vi "ArmPathPlannerDemo.vi"() -> ()   [LabVIEW 2018]
uses:
  OperatorControlBox_XControl.xctl
  TypeDefs/GamePiecePosition.ctl
  TypeDefs/ArmPositions.ctl
  TypeDefs/ArmAbsolutePosition.ctl
  TypeDefs/ArmPassThroughParams.ctl
  General/MotionProfiling/TypeDefs/MotionProfileGeneratorParams.ctl
  <vilib>/Rock Robotics/WPI/ThirdParty/Phoenix-LabVIEW/Motor Controller/Controls/CTRE_Phoenix_MotorControl_TrajectoryPointTimeDur.ctl
  TypeDefs/RobotID.ctl
  TypeDefs/ArmTargetPosition.ctl
  TypeDefs/JoystickControls.ctl
  TypeDefs/RobotComponents/RobotMotors.ctl
  <vilib>/Rock Robotics/WPI/MotorControl/WPI_MotorControlDeviceRef.ctl
  <vilib>/Rock Robotics/WPI/MotorControl/WPI_MotorControlType.ctl
  <vilib>/Rock Robotics/SystemInterfaces/DIO/FPGA_DIOPWMChannel.ctl
  <vilib>/Rock Robotics/WPI/PWM/WPI_PWMDeadband.ctl
  <vilib>/Rock Robotics/SystemInterfaces/DIO/FPGA_DIOChannel.ctl
  TypeDefs/ConfigComponents/Config_Robot.ctl
  ArgosLib/Config/ConfigComponents/TypeDefs/Config_Motor.ctl
  <vilib>/Rock Robotics/WPI/ThirdParty/Phoenix-LabVIEW/Motor Controller/Controls/CTRE_Phoenix_MotorControl_NeutralMode.ctl
  <vilib>/Rock Robotics/WPI/ThirdParty/Phoenix-LabVIEW/Motor Controller/Controls/CTRE_Phoenix_MotorControl_LimitSwitchNormal.ctl
  ArgosLib/Config/ConfigComponents/TypeDefs/Config_MotorCtrlType.ctl
  ArgosLib/Config/ConfigComponents/TypeDefs/Config_IMU.ctl
  <vilib>/Rock Robotics/SystemInterfaces/spilib/spi_bus.ctl
  ArgosLib/Config/ConfigComponents/TypeDefs/Config_DigitalIO.ctl
  ArgosLib/Config/ConfigComponents/TypeDefs/Config_PIDParams.ctl
  ArgosLib/Config/ConfigComponents/TypeDefs/Config_SingleSolenoid.ctl
  <vilib>/Rock Robotics/WPI/Solenoid/WPI_SolenoidChannel.ctl
  ArgosLib/Config/ConfigComponents/TypeDefs/Config_MotionMagicParams.ctl
  TypeDefs/ConfigComponents/Config_Dimensions.ctl
  TypeDefs/ArmCoordinate.ctl
  Climber/TypeDefs/ClimberPositionHeights.ctl
  General/MotionProfiling/TypeDefs/TrajectoryPoint.ctl
  ArgosLib/ArgosLib.lvlib
panel:
  in  "OutputTabControl":enum32{"Animation", "Path", "MotionProfiles"}(tab)
  out "Arm Position":cluster{"X":dbl[], "Y":dbl[]}[](graph)=[{"X"=[-15.5, -15.5, -7.0, -7.0, 7.0, 7.0, 15.5, 15.5, 45.5, 45.5, 7.0, 7.0, -7.0, -7.0, -45.5, -45.5, -15.5], "Y"=[0.0, 8.0, 8.0, 21.0, 21.0, 8.0, 8.0, 0.0, 0.0, 90.0, 90.0, 32.0, 32.0, 90.0, 90.0, 0.0, 0.0]}, {"X"=array[361 elements], "Y"=array[361 elements]}, {"X"=array[361 elements], "Y"=array[361 elements]}, {"X"=[0.0, 0.0], "Y"=[44.25, 26.0]}, {"X"=[0.0, 0.0], "Y"=[26.0, 20.0]}, {"X"=[0.0, -11.999996195182016, -11.999996195182016, 0.0], "Y"=[24.5, 24.4904440794712, 27.4904440794712, 27.5]}]
  out "Path":cluster{dbl[], dbl[]}[](graph)=[{array[361 elements], array[361 elements]}, {array[361 elements], array[361 elements]}, {[-15.5, -15.5, -7.0, -7.0, 7.0, 7.0, 15.5, 15.5, 45.5, 45.5, 7.0, 7.0, -7.0, -7.0, -45.5, -45.5, -15.5], [0.0, 8.0, 8.0, 21.0, 21.0, 8.0, 8.0, 0.0, 0.0, 90.0, 90.0, 32.0, 32.0, 90.0, 90.0, 0.0, 0.0]}, {[-12.5, -12.478433704418581, -12.402951669883615, -12.251987600813688, -12.003975201627373, -11.637348176743261, -11.141323378370641, -10.51590080650951, -9.761080461159862, -8.876862342321713, -7.863246449995051, -6.669969590682957, -5.189969590682963, -3.643302924016296, -2.05663625734963, -0.4566362573496323, 1.143363742650368, 2.7433637426503723, 4.343363742650376, 5.943363742650379, 7.542132189579336, 9.138056426829323, 10.733980664079322, 12.329904901329314, 13.925829138579315, 15.52175337582931, 17.117677613079312, 18.7136018503293, 20.309526087579293, 21.000000000000004, 20.999999999999996, 20.999999999999996, 20.999999999999993, 20.999999999999996, 21.000000000000004, 21.000000000000004, 21.000000000000004, 21.000000000000004, 21.000000000000004, 21.000000000000004, 21.000000000000004, 21.000000000000004, 21.000000000000004, 21.000000000000004], [17.0, 17.01568457860467, 17.07058060372101, 17.180372653953686, 17.36074530790737, 17.62738314418672, 17.988128452094085, 18.44298123162945, 18.99194148279283, 19.635009205584208, 20.372184400003597, 20.999999999999996, 21.0, 21.0, 21.0, 21.0, 21.0, 21.000000000000004, 20.999999999999996, 20.999999999999996, 21.038769982935307, 21.152900736713708, 21.267031490492112, 21.381162244270516, 21.49529299804892, 21.60942375182732, 21.72355450560572, 21.837685259384124, 21.951816013162524, 21.120098440989317, 19.613431774322653, 18.200098440989308, 16.90676510765598, 15.760098440989307, 15.0, 15.0, 15.0, 15.0, 15.0, 15.0, 15.0, 15.0, 15.0, 15.0]}]
  out "Overall Motion":T1(graph)={0.0, "Trajectory Point Interval (ms)"=40, [[0.0, 0.026666666666668868, 0.120000000000007, 0.30666666666667036, 0.6133333333333397, 1.0666666666666762, 1.6800000000000117, 2.4533333333333425, 3.386666666666679, 4.4800000000000075, 5.733333333333341, 7.081688661341715, 8.561688661341712, 10.108355328008379, 11.695021994675045, 13.295021994675043, 14.895021994675043, 16.495021994675046, 18.095021994675047, 19.695021994675052, 21.29426045671642, 22.894260456716413, 24.494260456716418, 26.094260456716416, 27.694260456716425, 29.294260456716426, 30.894260456716435, 32.49426045671643, 34.09426045671643, 35.1752361010282, 36.68190276769486, 38.095236101028206, 39.38856943436153, 40.535236101028204, 41.295334542017514, 41.295334542017514, 41.295334542017514, 41.295334542017514, 41.295334542017514, 41.295334542017514, 41.295334542017514, 41.295334542017514, 41.295334542017514, 41.295334542017514], [0.0, 0.6666666666667217, 2.3333333333334534, 4.666666666666584, 7.666666666666734, 11.333333333333412, 15.333333333333387, 19.333333333333268, 23.333333333333417, 27.333333333333208, 31.333333333333346, 33.70888320020935, 36.99999999999992, 38.66666666666667, 39.66666666666665, 39.99999999999994, 39.99999999999999, 40.00000000000008, 40.000000000000036, 40.00000000000012, 39.98096155103416, 39.99999999999986, 40.00000000000012, 39.99999999999994, 40.00000000000021, 40.000000000000036, 40.00000000000021, 39.99999999999994, 39.99999999999986, 27.024391107794266, 37.666666666666515, 35.333333333333705, 32.33333333333306, 28.666666666666885, 19.002461024732753, 0.0, 0.0, 0.0, 0.0, 0.0, 0.0, 0.0, 0.0, 0.0], [0.0, 16.666666666668043, 41.66666666666829, 58.33333333332828, 75.00000000000372, 91.66666666666696, 99.99999999999937, 99.99999999999702, 100.00000000000372, 99.99999999999476, 100.00000000000347, 59.38874667190008, 82.2779199947643, 41.66666666666874, 24.999999999999467, 8.333333333332327, 1.2434497875801753e-12, 2.1316282072803006e-12, -1.0658141036401503e-12, 2.1316282072803006e-12, -0.47596122414894637, 0.47596122414237385, 6.572520305780927e-12, -4.440892098500626e-12, 6.750155989720952e-12, -4.440892098500626e-12, 4.440892098500626e-12, -6.750155989720952e-12, -2.1316282072803006e-12, -324.3902223051398, 266.05688897180625, -58.33333333332025, -75.00000000001616, -91.66666666665435, -241.6051410483533, -475.0615256183188, 0.0, 0.0, 0.0, 0.0, 0.0, 0.0, 0.0, 0.0]]}
  out "Arm Shoulder":T1(graph)={0.0, "Trajectory Point Interval (ms)"=40, [[-0.43007813505586256, -0.4296420839132172, -0.42811056304482153, -0.4250223924235489, -0.4198751086410621, -0.41209365055679453, -0.40122632478789805, -0.3869398624770717, -0.36877462030765956, -0.34611168583234253, -0.3181268189017525, -0.2793774438131257, -0.219623853265813, -0.15543715949608483, -0.0882278321456805, -0.019637744370704407, 0.04913734990050419, 0.11745107310899316, 0.18468259919421834, 0.2502690642942215, 0.3141727633602416, 0.37673912272857585, 0.4369342229172807, 0.49448072535404136, 0.5491946894538539, 0.6009772159768075, 0.6498023221382211, 0.6957031748966047, 0.7387583479955007, 0.7371712252132288, 0.7058807841602786, 0.6784767269576032, 0.6549310323374246, 0.6351959881097435, 0.6226707887570674, 0.6226707887570674, 0.6226707887570674, 0.6226707887570674, 0.6226707887570674, 0.6226707887570674, 0.6226707887570674, 0.6226707887570674, 0.6226707887570674, 0.6226707887570674], [0.0, 0.010901278566134709, 0.03828802170989104, 0.07720426553181614, 0.12868209456217, 0.1945364521066889, 0.27168314422241213, 0.3571615577706591, 0.45413105423530303, 0.5665733618829257, 0.6996216732647511, 0.96873437721567, 1.4938397636828171, 1.604667344243204, 1.680233183760108, 1.7147521943744022, 1.7193773567802149, 1.7078430802122242, 1.6807881521306294, 1.6396616275000795, 1.5975924766505014, 1.5641589842083568, 1.5048775047176208, 1.4386625609190171, 1.3678491024953123, 1.294563163073842, 1.220627654035339, 1.1475213189595905, 1.0763793274723987, -0.03967806955679776, -0.782261026323755, -0.685101430066884, -0.5886423655044659, -0.4933761056920255, -0.3131299838169038, 0.0, 0.0, 0.0, 0.0, 0.0, 0.0, 0.0, 0.0, 0.0], [0.0, 0.2725319641533677, 0.6846685785939083, 0.9729060955481275, 1.2869457257588466, 1.6463589386129727, 1.9286673028930805, 2.1369603387061744, 2.424237411616098, 2.8110576911905674, 3.3262077845456344, 6.7278175987729725, 13.127634661678677, 2.770689514009672, 1.8891459879226025, 0.8629752653573519, 0.11562906014531693, -0.2883569141997666, -0.6763732020398705, -1.0281631157637472, -1.0517287712394519, -0.8358373110536166, -1.482036987268398, -1.6553735949650927, -1.7703364605926197, -1.832148485536761, -1.8483877259625747, -1.8276583768937094, -1.778549787179795, -27.901434925729912, -18.56457391917393, 2.4289899064217773, 2.411476614060451, 2.3816564953110104, 4.506153046878042, 7.828249595422595, 0.0, 0.0, 0.0, 0.0, 0.0, 0.0, 0.0, 0.0]]}
  out "Arm Extension":T1(graph)={0.0, "Trajectory Point Interval (ms)"=40, [[29.980201800521623, 29.956956524113412, 29.875643069970817, 29.713228111807556, 29.44702766897723, 29.05497549195633, 28.527442644235364, 27.86729960874173, 27.078556309890278, 26.16670512031852, 25.139226769349754, 24.187827400174566, 23.822222489772315, 23.533723806404836, 23.34078517734665, 23.25448379714171, 23.27809658558894, 23.411290964500196, 23.652215722865584, 23.997626394655185, 24.405838581580717, 24.839083510428015, 25.366024174195292, 25.980960243487978, 26.67780740506135, 27.450328244110118, 28.292324638976435, 29.19778666688754, 30.160998972396772, 31.24087620617458, 32.37221793356851, 33.460385102896645, 34.47683997088334, 35.393141861695746, 36.007811652473414, 36.007811652473414, 36.007811652473414, 36.007811652473414, 36.007811652473414, 36.007811652473414, 36.007811652473414, 36.007811652473414, 36.007811652473414, 36.007811652473414], [0.0, -0.5811319102052792, -2.032836353564882, -4.06037395408152, -6.655011070758121, -9.801304425522517, -13.188321193024155, -16.503575887340816, -19.71858247128635, -22.7962797392939, -25.686958774219182, -23.784984229379713, -9.140122760056268, -7.212467084186969, -4.823465726454668, -2.157534505123504, 0.5903197111807756, 3.3298594727813935, 6.023118959134699, 8.635266794740026, 10.205304673138293, 10.831123221182448, 13.173516594181933, 15.373401732317138, 17.421179039334334, 19.313020976219164, 21.049909871657935, 22.636550697777658, 24.08030763773077, 26.99693084444519, 28.28354318484818, 27.20417923320344, 25.411371699667384, 22.907547270310147, 15.36674476944171, 0.0, 0.0, 0.0, 0.0, 0.0, 0.0, 0.0, 0.0, 0.0], [0.0, -14.52829775513198, -36.29261108399007, -50.68844001291595, -64.86592791691503, -78.65733386910989, -84.67541918754095, -82.88136735791652, -80.37516459863836, -76.94243170018878, -72.26697587313203, 47.54936362098672, 366.1215367330861, 48.19139189673249, 59.72503394330752, 66.64828053327909, 68.69635540760699, 68.48849404001544, 67.33148715883263, 65.30369589013318, 39.25094695995668, 15.645463701103868, 58.55983432498712, 54.997128453380114, 51.19443267542989, 47.29604842212076, 43.42222238596926, 39.66602065299307, 36.093923498827785, 72.91558016786048, 32.165308510074816, -26.984098791118516, -44.8201883384014, -62.59561073393094, -188.52006252171094, -384.16861923604273, 0.0, 0.0, 0.0, 0.0, 0.0, 0.0, 0.0, 0.0]]}
  out "Arm Wrist":T1(graph)={0.0, "Trajectory Point Interval (ms)"=40, [[-1.1399218649441374, -1.1401271167743305, -1.140850840049144, -1.14132230153005, -1.1365047811265363, -1.1178912992924164, -1.0702017132109638, -0.9734500998505116, -0.801776128514992, -0.5257829978420447, -0.10845271313207694, 0.27973404246175215, 0.22672620863261558, 0.178875608022439, 0.1383139859985968, 0.1067322525928331, 0.0851051506059308, 0.07415682103779947, 0.07441631260600232, 0.08653187322417216, 0.1104806304708435, 0.1459394874228916, 0.19394990462002182, 0.2547512366794354, 0.3285998292366029, 0.4155054833836992, 0.5155822451523272, 0.6287266123351376, 0.7548959253420735, 0.8328287747867713, 0.8641192158397215, 0.8915232730423969, 0.9150689676625755, 0.9348040118902565, 0.9473292112429327, 0.9473292112429327, 0.9473292112429327, 0.9473292112429327, 0.9473292112429327, 0.9473292112429327, 0.9473292112429327, 0.9473292112429327, 0.9473292112429327, 0.9473292112429327], [0.0, -0.005131295754828846, -0.018093081870335093, -0.011786537022651089, 0.12043801008784216, 0.4653370458529982, 1.1922396520363143, 2.4187903340113057, 4.291849283387989, 6.899828266823682, 10.433257117749195, 9.704668889845728, -1.3251958457284143, -1.196265015254415, -1.014040550596055, -0.7895433351440921, -0.5406775496725577, -0.27370823920328313, 0.006487289205071162, 0.3028890154542461, 0.5987189311667834, 0.8864714238012023, 1.2002604299282558, 1.5200333014853393, 1.846214813929188, 2.172641353677407, 2.5019190442157, 2.82860917957026, 3.1542328251733975, 1.9483212361174451, 0.782261026323755, 0.685101430066884, 0.5886423655044659, 0.4933761056920255, 0.3131299838169038, 0.0, 0.0, 0.0, 0.0, 0.0, 0.0, 0.0, 0.0, 0.0], [0.0, -0.12828239387072116, -0.32404465288765616, 0.1576636211921001, 3.3056136777623313, 8.6224758941289, 18.1725651545829, 30.663767049374783, 46.82647373441707, 65.19947458589232, 88.33572127313782, -18.214705697586673, -275.74661838935356, 3.2232707618499834, 4.555611616458998, 5.612430386299072, 6.221644636788362, 6.674232761731863, 7.004888210208857, 7.410043156229373, 7.395747892813432, 7.1938123158604705, 7.844725153176338, 7.994321788927089, 8.154537811096219, 8.160663493705473, 8.231942263457325, 8.167253383864004, 8.140591140078435, -30.14778972639881, -29.15150524484225, -2.4289899064217773, -2.411476614060451, -2.3816564953110104, -4.506153046878042, -7.828249595422595, 0.0, 0.0, 0.0, 0.0, 0.0, 0.0, 0.0, 0.0]]}
  in  "InputTabControl":T2(tab)
  in  "stop":bool
  in  "OperatorControlBox":cluster{"OperatorControlBox Buttons":T3}(xcontrol)={"OperatorControlBox Buttons"={"Position_FeederStation"=FALSE, "Position_Depot"=FALSE, "Position_NearRocket_Low"=FALSE, "Position_NearRocket_Mid"=FALSE, "Position_NearRocket_High"=FALSE, " Position_FarRocket_Low"=FALSE, "Position_FarRocket_Mid"=FALSE, "Position_FarRocket_High"=FALSE, "Mode_Hatch"=FALSE, "Mode_Cargo"=TRUE, "Side_Left"=TRUE, "Side_Right"=FALSE, "Climb"=FALSE, "Switch1_Left"=TRUE, "Switch1_Right"=FALSE, "Switch2_Left"=TRUE, "Switch2_Right"=FALSE, "Button1"=FALSE, "Button2"=FALSE, "Button3"=FALSE, "Button4"=FALSE, "Position_CargoShip"=FALSE}}
  in  "Game Piece Position":T4={"Hatch Forward"={"FeederStation"={"X (in)"=13.0, "Y (in)"=18.0, "Wrist (rad)"=1.8}, "Low"={"X (in)"=14.0, "Y (in)"=19.0, "Wrist (rad)"=1.7}, "Mid"={"X (in)"=16.0, "Y (in)"=52.0, "Wrist (rad)"=1.57}, "High"={"X (in)"=11.0, "Y (in)"=75.0, "Wrist (rad)"=1.57}, "FloorIntake"={"X (in)"=-12.5, "Y (in)"=17.0, "Wrist (rad)"=-1.57}, "CargoShip"={"X (in)"=9.0, "Y (in)"=19.0, "Wrist (rad)"=1.8}}, "Hatch Reverse"={"FeederStation"={"X (in)"=-16.0, "Y (in)"=24.0, "Wrist (rad)"=-1.57}, "Low"={"X (in)"=-15.0, "Y (in)"=23.0, "Wrist (rad)"=-1.75}, "Mid"={"X (in)"=-16.0, "Y (in)"=52.0, "Wrist (rad)"=-1.57}, "High"={"X (in)"=-9.0, "Y (in)"=79.0, "Wrist (rad)"=-1.7}, "FloorIntake"={"X (in)"=-12.5, "Y (in)"=17.0, "Wrist (rad)"=-1.57}, "CargoShip"={"X (in)"=-11.0, "Y (in)"=24.0, "Wrist (rad)"=-1.57}}, "Cargo Forward"={"FeederStation"={"X (in)"=-12.5, "Y (in)"=17.0, "Wrist (rad)"=-1.57}, "Low"={"X (in)"=13.0, "Y (in)"=32.0, "Wrist (rad)"=2.2}, "Mid"={"X (in)"=9.0, "Y (in)"=60.0, "Wrist (rad)"=2.2}, "High"={"X (in)"=12.0, "Y (in)"=70.0, "Wrist (rad)"=1.57}, "FloorIntake"={"X (in)"=21.0, "Y (in)"=15.0, "Wrist (rad)"=1.57}, "CargoShip"={"X (in)"=16.0, "Y (in)"=52.0, "Wrist (rad)"=1.57}}, "Cargo Reverse"={"FeederStation"={"X (in)"=-16.0, "Y (in)"=25.5, "Wrist (rad)"=-1.57}, "Low"={"X (in)"=-16.0, "Y (in)"=25.5, "Wrist (rad)"=-1.2}, "Mid"={"X (in)"=-16.0, "Y (in)"=52.0, "Wrist (rad)"=-1.2}, "High"={"X (in)"=-9.0, "Y (in)"=78.0, "Wrist (rad)"=-1.4}, "FloorIntake"={"X (in)"=-18.0, "Y (in)"=15.0, "Wrist (rad)"=0.0}, "CargoShip"={"X (in)"=-18.0, "Y (in)"=50.0, "Wrist (rad)"=-1.0}}, "Hold"={"X (in)"=0.0, "Y (in)"=26.0, "Wrist (rad)"=0.0}}
  in  "Arm MotionProfileParams":T7={"Trajectory Point Interval (ms)"=40, "Maximum Travel Speed (units/s)"=40.0, "Velocity Ramp Time (ms)"=400.0, "Acceleration Ramp Time (ms)"=200.0} {"Acceleration Ramp Time (ms)" min=1.0; "Velocity Ramp Time (ms)" min=1.0; "Maximum Travel Speed (units/s)" min=0.0; "Trajectory Point Interval (ms)" items=["TrajectoryDuration_0ms"=0, "TrajectoryDuration_5ms"=5, "TrajectoryDuration_10ms"=10, "TrajectoryDuration_20ms"=20, "TrajectoryDuration_30ms"=30, "TrajectoryDuration_40ms"=40, "TrajectoryDuration_50ms"=50, "TrajectoryDuration_100ms"=100]}
  in  "Arm Pass Through Params":T9={"Pass Through Length (in)"=14.0, "Pass Through Min Height (in)"=21.0, "Pass Through Max Height (in)"=32.0, "Pass Through Wrist Angle (rad)"=0.0}
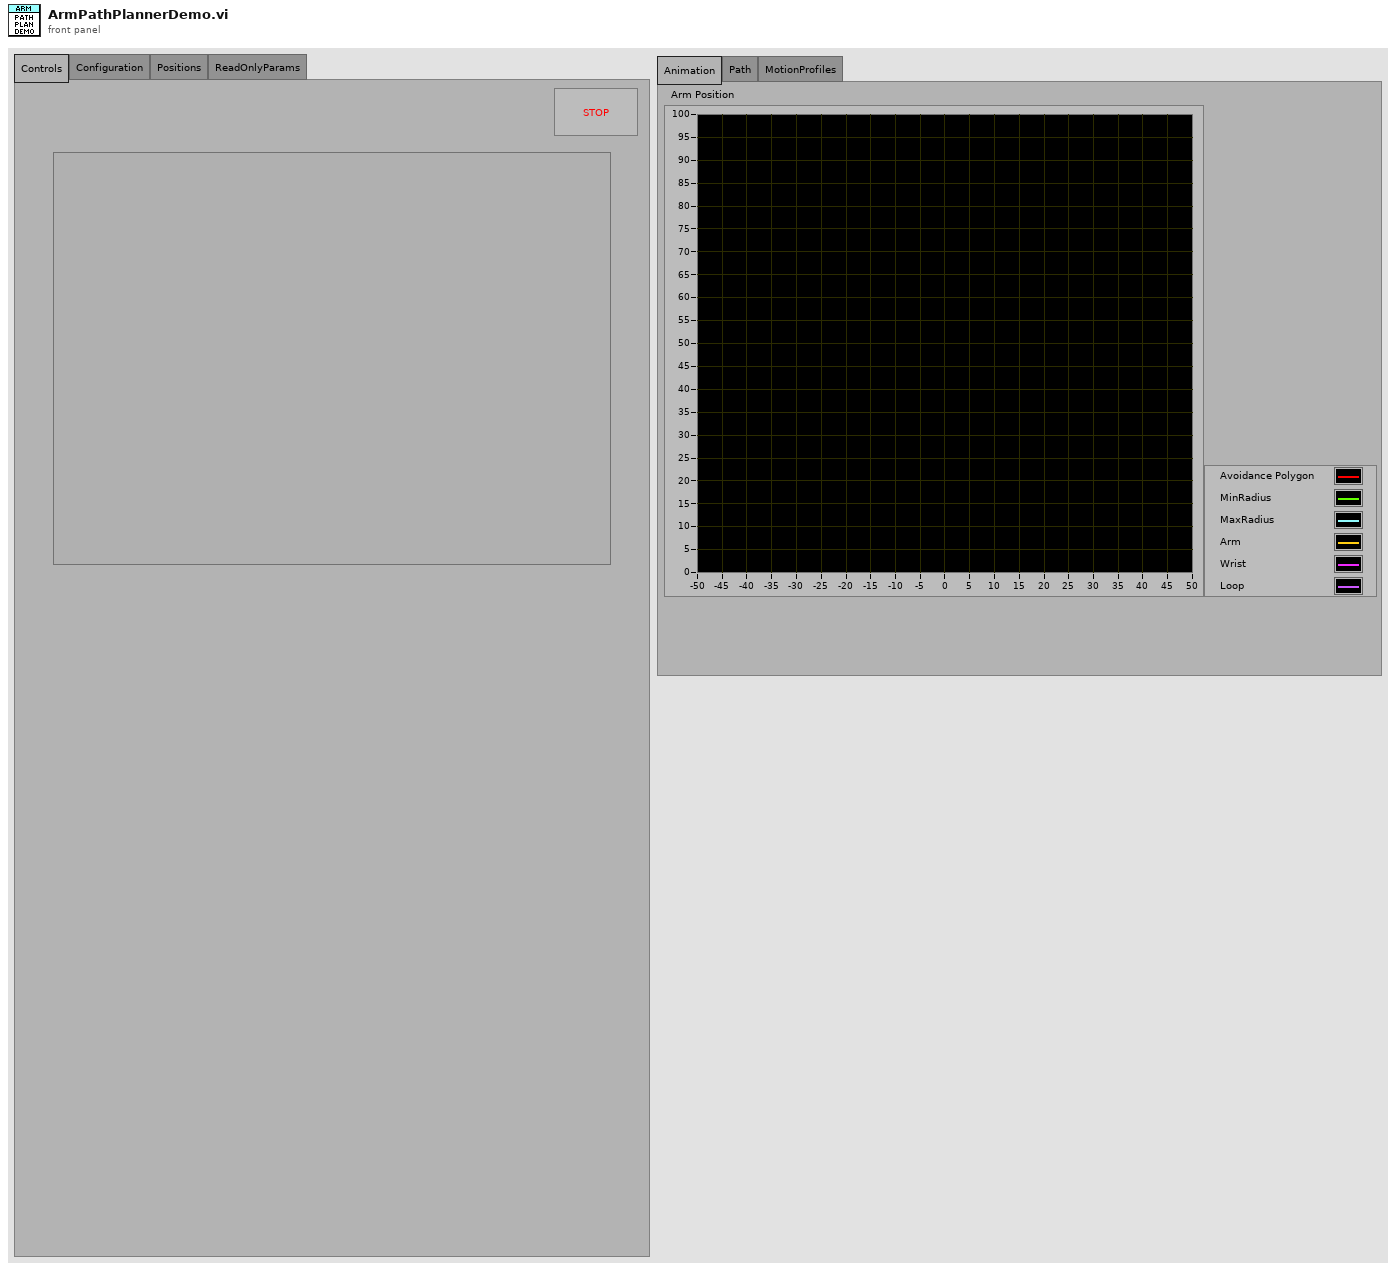
[diagram p1: front panel]
types:
  T1 = cluster{dbl, "Trajectory Point Interval (ms)":i32, dbl[][]}
  T2 = enum32{"Controls", "Configuration", "Positions", "ReadOnlyParams"}
  T3 = typedef "OperatorControlBoxButtons_Type.ctl" = cluster{"Position_FeederStation":bool, "Position_Depot":bool, "Position_NearRocket_Low":bool, "Position_NearRocket_Mid":bool, "Position_NearRocket_High":bool, " Position_FarRocket_Low":bool, "Position_FarRocket_Mid":bool, "Position_FarRocket_High":bool, "Mode_Hatch":bool, "Mode_Cargo":bool, "Side_Left":bool, "Side_Right":bool, "Climb":bool, "Switch1_Left":bool, "Switch1_Right":bool, "Switch2_Left":bool, "Switch2_Right":bool, "Button1":bool, "Button2":bool, "Button3":bool, "Button4":bool, "Position_CargoShip":bool}
  T4 = typedef "GamePiecePosition.ctl" = cluster{"Hatch Forward":T5, "Hatch Reverse":T5, "Cargo Forward":T5, "Cargo Reverse":T5, "Hold":T6}
  T5 = typedef "ArmPositions.ctl" = cluster{"FeederStation":T6, "Low":T6, "Mid":T6, "High":T6, "FloorIntake":T6, "CargoShip":T6}
  T6 = typedef "ArmAbsolutePosition.ctl" = cluster{"X (in)":dbl, "Y (in)":dbl, "Wrist (rad)":dbl}
  T7 = typedef "MotionProfileGeneratorParams.ctl" = cluster{"Trajectory Point Interval (ms)":T8, "Maximum Travel Speed (units/s)":dbl, "Velocity Ramp Time (ms)":dbl, "Acceleration Ramp Time (ms)":dbl}
  T8 = typedef "CTRE_Phoenix_MotorControl_TrajectoryPointTimeDur.ctl" = i32
  T9 = typedef "ArmPassThroughParams.ctl" = cluster{"Pass Through Length (in)":dbl, "Pass Through Min Height (in)":dbl, "Pass Through Max Height (in)":dbl, "Pass Through Wrist Angle (rad)":dbl}
  T10 = typedef "JoystickControls.ctl" = cluster{"Drive":dbl, "Drive Turn ":dbl, "Unassigned_LX":dbl, "Unassigned_RY":dbl, "Claw Release":bool, "Place":dbl, "Feeder":dbl, "SP Low":bool, "SP Mid":bool, "SP High":bool, "Shift":bool, "Arm Go To Position":bool, "Unassigned_LJ":bool, "Unassigned_RJ":bool, "Swap_Back":bool, "Swap_Start":bool, "Unassigned_LY 2":dbl, "Unassigned_RX 2":dbl, "Unassigned_LX 2":dbl, "Unassigned_RY 2":dbl, "SP Feeder Station":bool, "Back Intake REV":dbl, "Front Intake REV":dbl, "SP Low 2":bool, "SP Mid 2":bool, "SP High 2":bool, "Hatch/Cargo":bool, "Go to Hold":bool, "Unassigned_LJ 2":bool, "Unassigned_RJ 2":bool, "Swap_Back 2":bool, "Swap_Start 2":bool, "Unassigned_Up 2":bool, "Unassigned_Right 2":bool, "Arm Return":bool, "Unassigned_Left 2":bool, "Auto Climb":bool, " Unassigned_Right":bool, "Unassigned_Down":bool, "Unassigned_Left":bool, "Shoulder":dbl, "Unassigned_RX 3":dbl, "Unassigned_LX 3":dbl, "Arm Extend":dbl, "Climb Drive Reverse":bool, "Wrist CCW":dbl, "Wrist CW":dbl, "Rev Intake Extend":bool, "Fw Intake Extend":bool, "Climb Dr Forward":bool, "Intake Ingest ":bool, "Claw Release 3":bool, "Unassigned_LJ 3":bool, "Unassigned_RJ 3":bool, "Intake Puke":bool, "Unassigned Start 3":bool, "Climb F Up":bool, "Climb R Up":bool, "Climb F Down":bool, "Climb R Down":bool}
  T11 = typedef "ArmTargetPosition.ctl" = enum16{"Forward Cargo Floor Intake", "Forward Cargo Feeder Station", "Forward Cargo Low", "Forward Cargo Middle", "Forward Cargo High", "Forward Cargo CargoShip", "Forward Hatch Floor Intake", "Forward Hatch Feeder Station", "Forward Hatch Low", "Forward Hatch Middle", "Forward Hatch High", "Forward Hatch CargoShip", "Reverse Cargo Floor Intake", "Reverse Cargo Feeder Station", "Reverse Cargo Low", "Reverse Cargo Middle", "Reverse Cargo High", "Reverse Cargo CargoShip", "Reverse Hatch Floor Intake", "Reverse Hatch Feeder Station", "Reverse Hatch Low", "Reverse Hatch Middle", "Reverse Hatch High", "Reverse Hatch CargoShip", "Hold"}
  T12 = typedef "RobotID.ctl" = enum16{"Competition", "Practice", "Programming"}
  T13 = typedef "TrajectoryPoint.ctl" = cluster{"Position ":dbl, "Velocity ":dbl, "Time (ms)":T8, "Last Point":bool}
  T14 = typedef "Config_Robot.ctl" = cluster{"Motors":cluster{"DriveRightPrimary":T15, "DriveRightSecondary":T15, "DriveLeftPrimary":T15, "DriveLeftSecondary":T15, "RearClimb":T15, "Front Climb":T15, "Climb Drive":T15, "Shoulder1":T15, "Shoulder2":T15, "Wrist":T15, "Extension":T15, "CargoIntake":T15, "Intake2":T15}, "Sensors":cluster{"IMU":T20, "HomingButton":T22, "HomingLED_Green":T22, "HomingLED_Yellow":T22, "HomingLED_Red":T22}, "PID":cluster{"FrontClimb":T24, "RearClimb":T24, "ArmShoulder":T24, "ArmExtend":T24, "ArmWrist":T24}, "Solenoids":cluster{" Shifter":T25, "Hatch Grip":T25, "Hatch Extend":T25, "Manipulator Slide":T25, "Hatch Floor Intake":T25}, "Enable Compressor":bool, "MotionMagic":cluster{"FrontClimbExtend":T27, "RearClimbExtend":T27, "FrontClimbRetract":T27, "RearClimbRetract":T27}, "RobotDimensions":T28, "Arm Home Position":T29, "Climb Home Position":cluster{"Back Climb":dbl, "Front Climb":dbl}, "Climb Positions":T30}
  T15 = typedef "ArgosLib.lvlib/Config_Motor.ctl" = cluster{"CAN Address":u8, "Invert":bool, "InvertSensor":bool, "Unit Conversion Factor":dbl, "Brake Mode":T16, "Reverse Limt Switch Mode":T17, "Forward Limt Swith Mode":T17, "PWM Channel":T18, "Motor Controller Type":T19, "Peak Current (A)":i32, "Continuos Current (A)":i32, "Peak Duration (ms)":i32, "Current Limit Enable":bool}
  T16 = typedef "CTRE_Phoenix_MotorControl_NeutralMode.ctl" = enum8{"EEPROMSetting", "Override to Coast", "Override to Brake"}
  T17 = typedef "CTRE_Phoenix_MotorControl_LimitSwitchNormal.ctl" = enum16{"Normally Open", "Normally Closed", "Disabled"}
  T18 = typedef "FPGA_DIOPWMChannel.ctl" = enum8{"PWM 0", "PWM 1", "PWM 2", "PWM 3", "PWM 4", "PWM 5", "PWM 6", "PWM 7", "PWM 8", "PWM 9", "PWM MXP 0", "PWM MXP 1", "PWM MXP 2", "PWM MXP 3", "PWM MXP 4", "PWM MXP 5", "PWM MXP 6", "PWM MXP 7", "PWM MXP 8", "PWM MXP 9", "Invalid"}
  T19 = typedef "ArgosLib.lvlib/Config_MotorCtrlType.ctl" = enum16{"Disabled", "Talon SRX", "Talon SR"}
  T20 = typedef "ArgosLib.lvlib/Config_IMU.ctl" = cluster{"Yaw Axis":enum16{"X", "Y", "Z"}, "SPI Bus":T21, "AHRS Algorithm":enum16{"Complementary", "Madgwick"}, "Calibration Time (s)":dbl, "Calibrate On Open":bool}
  T21 = typedef "spi_bus.ctl" = enum16{"SPI On-Board, CS0", "SPI On-Board, CS1", "SPI On-Board, CS2", "SPI On-Board, CS3", "SPI MXP", "Invalid"}
  T22 = typedef "ArgosLib.lvlib/Config_DigitalIO.ctl" = cluster{"DIOChannel":T23, "Active Low":bool}
  T23 = typedef "FPGA_DIOChannel.ctl" = enum8{"DIO 0", "DIO 1", "DIO 2", "DIO 3", "DIO 4", "DIO 5", "DIO 6", "DIO 7", "DIO 8", "DIO 9", "DIO MXP 0", "DIO MXP 1", "DIO MXP 2", "DIO MXP 3", "DIO MXP 4", "DIO MXP 5", "DIO MXP 6", "DIO MXP 7", "DIO MXP 8", "DIO MXP 9", "DIO MXP 10", "DIO MXP 11", "DIO MXP 12", "DIO MXP 13", "DIO MXP 14", "DIO MXP 15", "SPI Port CS1", "SPI Port CS2", "SPI Port CS3", "SPI Port MISO", "SPI Port MOSI", "Invalid"}
  T24 = typedef "ArgosLib.lvlib/Config_PIDParams.ctl" = cluster{"P":dbl, "I":dbl, "D":dbl, "F":dbl, "IZone":dbl}
  T25 = typedef "ArgosLib.lvlib/Config_SingleSolenoid.ctl" = cluster{"SolenoidChannel":T26, "Invert":bool}
  T26 = typedef "WPI_SolenoidChannel.ctl" = enum8{"Solenoid 0", "Solenoid 1", "Solenoid 2", "Solenoid 3", "Solenoid 4", "Solenoid 5", "Solenoid 6", "Solenoid 7", "Invalid"}
  T27 = typedef "Config_MotionMagicParams.ctl" = cluster{"CruiseVelocity":i32, "Acceleration":i32}
  T28 = typedef "Config_Dimensions.ctl" = cluster{"Length (in)":dbl, "Shoulder Height (in)":dbl, "Frame Height (in)":dbl, "Arm Center to Front of Robot (in)":dbl, "Arm Min Extension (in)":dbl, "Arm Max Extension (in)":dbl, "Cargo Intake Loop Length (in)":dbl, "Cargo Intake Loop Width (in)":dbl, "Cargo Intake Loop Offset (in)":dbl, "Cargo Intake Loop Angle (rad)":dbl}
  T29 = typedef "ArmCoordinate.ctl" = cluster{"Radius (in)":dbl, "ShoulderAngle (rad)":dbl, "WristAngle (rad)":dbl}
  T30 = typedef "ClimberPositionHeights.ctl" = cluster{"Retract":dbl, "Level 2":dbl, "Level 3":dbl}
  T31 = typedef "RobotMotors.ctl" = cluster{"DriveRightPrimary":T32, "DriveRightSecondary":T32, "DriveLeftPrimary":T32, "DriveLeftSecondary":T32, " RearClimb":T32, "FrontClimb":T32, "ClimbDrive":T32, "Shoulder2":T32, "Shoulder1 ":T32, "Wrist":T32, "Extension":T32, "CargoIntake":T32, "Intake2":T32}
  T32 = typedef "WPI_MotorControlDeviceRef.ctl" = cluster{"DeviceStatus":errorcluster, "Type":T33, "PWM":cluster{"PWM Channel":T18, "DeadBand":T34}, "CAN":cluster{"Device Number":u8, "SetOutput VI Ref":variant, "GetOutput VI Ref":variant, "Enable VI Ref":variant, "Disable VI Ref":variant, "Data":variant}, "Invert":bool, "DIO PWM":cluster{"PWM \"Enable\" Channel":T18, "DIOChannel":T23, "PWM Rate":dbl}}
  T33 = typedef "WPI_MotorControlType.ctl" = enum16{"PWM", "CAN", "DIO PWM"}
  T34 = typedef "WPI_PWMDeadband.ctl" = cluster{"Name":string, "maxPositivePwm":i32, "minPositivePwm":i32, "centerPwm":i32, "maxNegativePwm":i32, "minNegativePwm":i32, "angularRange":u16}
  T35 = typedef "ArgosLib.lvlib/Polygon2D.ctl" = T36[]
  T36 = typedef "ArgosLib.lvlib/Point2D.ctl" = cluster{"X (in)":dbl, "Y (in)":dbl}
  T37 = typedef "ArmPlanRequest.ctl" = cluster{"Destination":T11, "Preview":bool, "Start":T11, "Fixed Start":bool}
  T38 = typedef "ArmPlanResponse.ctl" = cluster{"ShoulderTrajectory":T13[], "ExtendTrajectory":T13[], "PlanTime (ms)":u32, "Execute":bool, "WristTrajectory":T13[]}
  T39 = cluster{dbl, "Trajectory Point Interval (ms)":T8, dbl[][]}
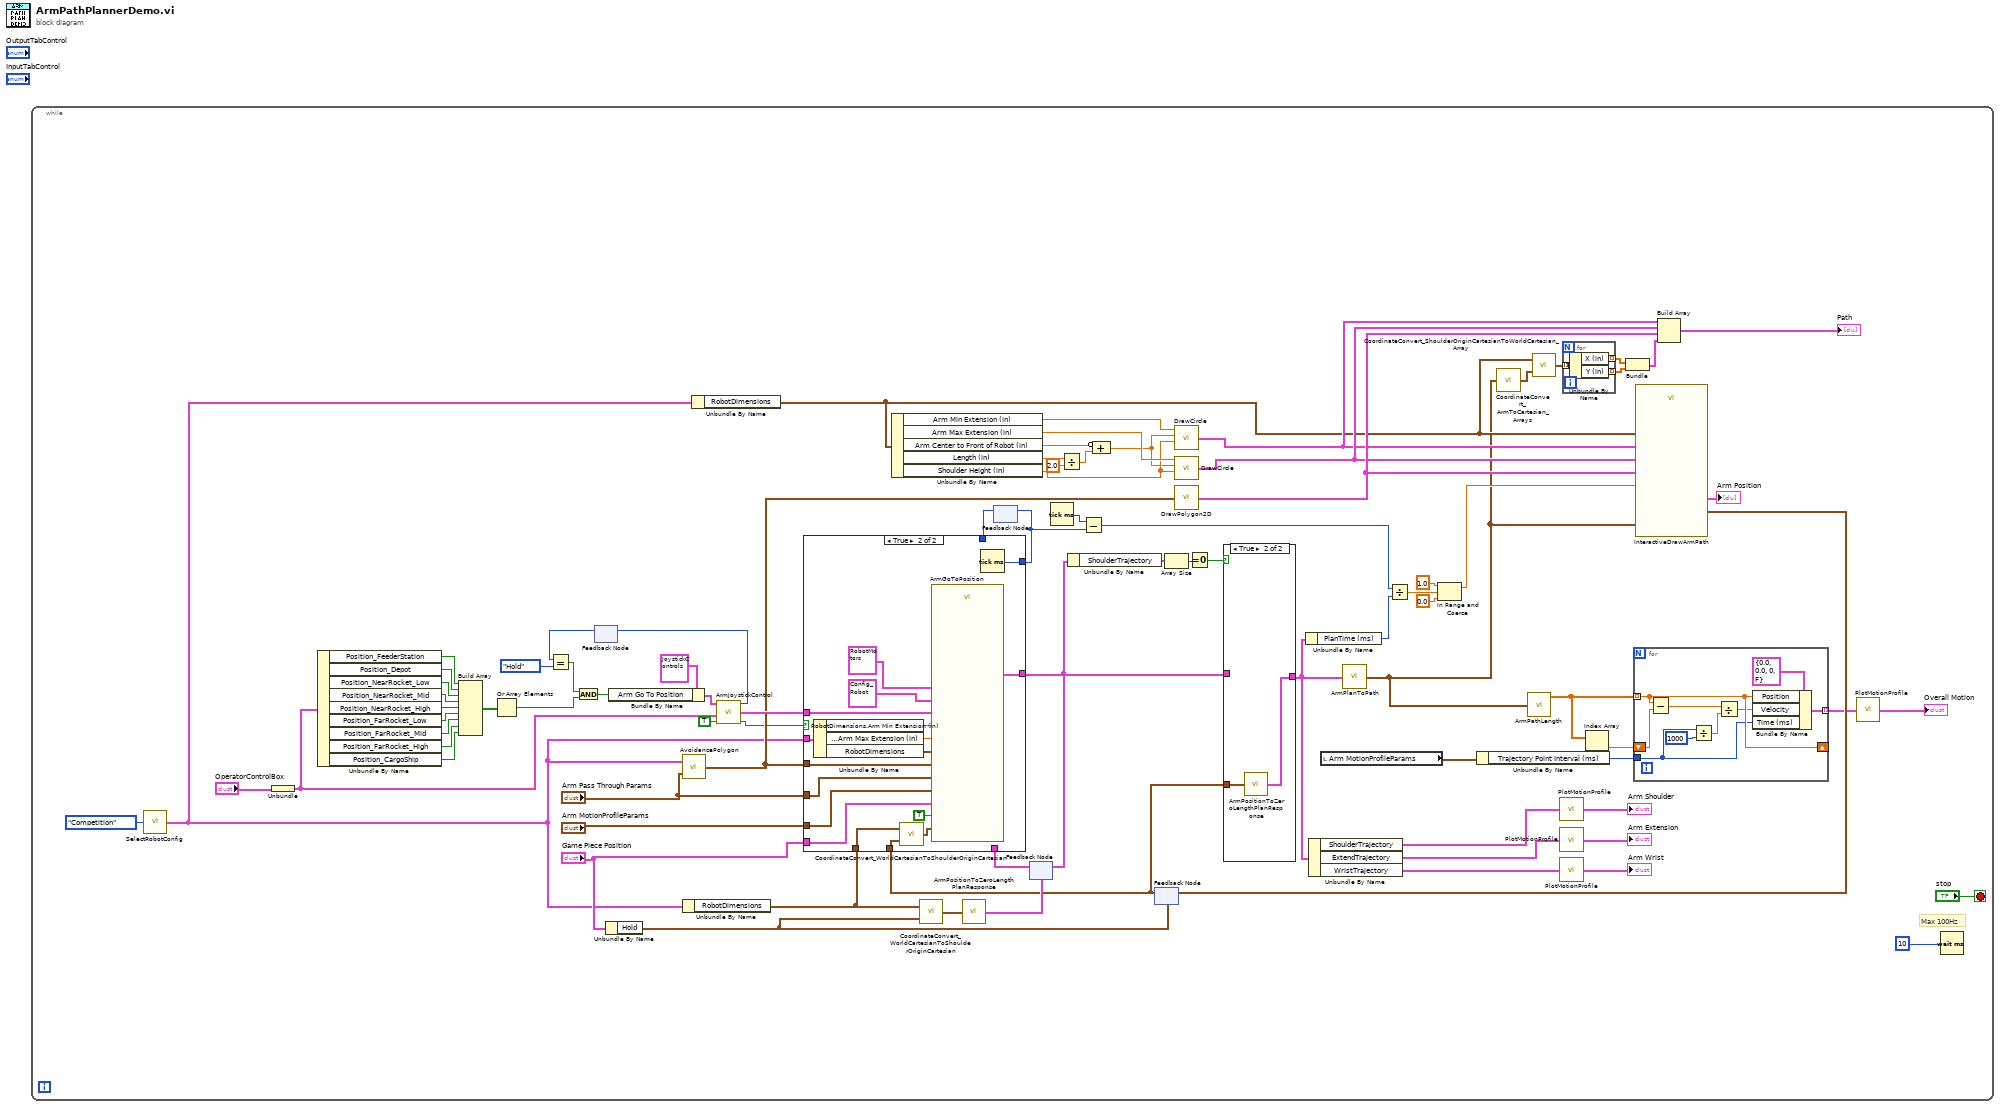
[diagram p0: block diagram]
diagram:
  n1 = while {
    stop <- "stop" stop-if-true
    # "Max 100Hz"
    n2 = call "SelectRobotConfig.vi"("Robot ID"=RobotID."Competition") -> ("Selected Config"=w28:T14)
    n3 = Unbundle("OperatorControlBox") -> ("OperatorControlBox Buttons"=w77:T3)
    n4 = Unbundle By Name(w77) -> ("Position_FeederStation"=w76:bool, "Position_Depot"=w75:bool, "Position_NearRocket_Low"=w74:bool, "Position_NearRocket_Mid"=w73:bool, "Position_NearRocket_High"=w72:bool, "Position_FarRocket_Low"=w71:bool, "Position_FarRocket_Mid"=w70:bool, "Position_FarRocket_High"=w69:bool, "Position_CargoShip"=w68:bool)
    n5 = Build Array(w76, w75, w74, w73, w72, w71, w70, w69, w68) -> (w67:bool[])
    n6 = Or Array Elements(Boolean array=w67) -> (logical OR=w65:bool)
    n7 = feedback #1() -> (w79:T11)  [unwired: 1 in]
    n8 = Equal?(x=w79, y=ArmTargetPosition."Hold") -> (x = y?=w66:bool)
    n9 = And(x=w66, y=w65) -> (x .and. y?=w62:bool)
    n10 = Unbundle By Name("Game Piece Position") -> ("Hold"=w30:T6)
    n11 = Bundle By Name(cluster=T10 {"Drive"=0.0, "Drive Turn "=0.0, "Unassigned_LX"=0.0, "Unassigned_RY"=0.0, "Claw Release"=FALSE, "Place"=0.0, "Feeder"=0.0, "SP Low"=FALSE, "SP Mid"=FALSE, "SP High"=FALSE, "Shift"=FALSE, "Arm Go To Position"=FALSE, "Unassigned_LJ"=FALSE, "Unassigned_RJ"=FALSE, "Swap_Back"=FALSE, "Swap_Start"=FALSE, "Unassigned_LY 2"=0.0, "Unassigned_RX 2"=0.0, "Unassigned_LX 2"=0.0, "Unassigned_RY 2"=0.0, "SP Feeder Station"=FALSE, "Back Intake REV"=0.0, "Front Intake REV"=0.0, "SP Low 2"=FALSE, "SP Mid 2"=FALSE, "SP High 2"=FALSE, "Hatch/Cargo"=FALSE, "Go to Hold"=FALSE, "Unassigned_LJ 2"=FALSE, "Unassigned_RJ 2"=FALSE, "Swap_Back 2"=FALSE, "Swap_Start 2"=FALSE, "Unassigned_Up 2"=FALSE, "Unassigned_Right 2"=FALSE, "Arm Return"=FALSE, "Unassigned_Left 2"=FALSE, "Auto Climb"=FALSE, " Unassigned_Right"=FALSE, "Unassigned_Down"=FALSE, "Unassigned_Left"=FALSE, "Shoulder"=0.0, "Unassigned_RX 3"=0.0, "Unassigned_LX 3"=0.0, "Arm Extend"=0.0, "Climb Drive Reverse"=FALSE, "Wrist CCW"=0.0, "Wrist CW"=0.0, "Rev Intake Extend"=FALSE, "Fw Intake Extend"=FALSE, "Climb Dr Forward"=FALSE, "Intake Ingest "=FALSE, "Claw Release 3"=FALSE, "Unassigned_LJ 3"=FALSE, "Unassigned_RJ 3"=FALSE, "Intake Puke"=FALSE, "Unassigned Start 3"=FALSE, "Climb F Up"=FALSE, "Climb R Up"=FALSE, "Climb F Down"=FALSE, "Climb R Down"=FALSE} ("Joystick control"), "Arm Go To Position"=w62) -> (w63:T10)
    n12 = call "AvoidancePolygon.vi"("Arm Pass Through Params"="Arm Pass Through Params", "RobotConfig"=w28) -> ("Polygon"=w55:T35)
    n13 = Unbundle By Name(w28) -> ("RobotDimensions"=w26:T28)
    n14 = Unbundle By Name(w28) -> ("RobotDimensions"=w22:T28)
    n15 = call "ArmJoystickControl.vi"("OperatorControlBox Enable"=TRUE, "OperatorControlBox Buttons"=w77, "Joystick control"=w63) -> ("NewPath"=w46:bool, "ArmPlanRequest"=w61:T37, "TargetPosition"=w80:T11)  [unwired: 1 in, 1 out]
    n16 = feedback-in #1(w80) -> ()
    n17 = Unbundle By Name(w22) -> ("Arm Min Extension (in)"=w54:dbl, "Arm Max Extension (in)"=w53:dbl, "Arm Center to Front of Robot (in)"=w48:dbl, "Length (in)"=w52:dbl, "Shoulder Height (in)"=w50:dbl)
    n18 = call "CoordinateConvert_WorldCartesianToShoulderOriginCartesian.vi"("ArmPositionIn"=w30, "RobotDimensions"=w26) -> ("ArmPositionRelativeToShoulder"=w29:T6)
    n19 = call "ArmPositionToZeroLengthPlanResponse.vi"("Position"=w29) -> ("ArmPlanResponse"=w40:T38)
    n20 = feedback #2() -> (w39:u32)  [unwired: 1 in]
    n21 = feedback #3(w40) -> (w45:T38)
    n22 = Tick Count (ms)() -> (millisecond timer value=w38:u32)
    n23 = Divide(x=w52, y=2.0) -> (x/y=w49:dbl)
    n24 = Compound Arithmetic op=ADD(invert w48, w49) -> (w47:dbl)
    n25 = feedback #4(w30) -> (w27:T6)
    n26 = case shown="True" w46 {
      tunnel: w61 -> [_ w118]
      tunnel: "Arm MotionProfileParams" -> [_ w114]
      tunnel: "Arm Pass Through Params" -> [_ w113]
      tunnel: "Game Piece Position" -> [_ w109]
      tunnel: w55 -> [_ w108]
      tunnel: w28 -> [_ w107]
      tunnel: [w101 w106] -> w41
      tunnel: w45 -> [w101 _]
      tunnel: [w100 w105] -> w37
      tunnel: w39 -> [w100 _]
      tunnel: w27 -> [_ w103]
      tunnel: w26 -> [_ w102]
      frame False {
      }
      frame True {
        n27 = Unbundle By Name(w107) -> ("RobotDimensions.Arm Min Extension (in)"=w112:dbl, "RobotDimensions.Arm Max Extension (in)"=w111:dbl, "RobotDimensions"=w110:T28)
        n28 = call "CoordinateConvert_WorldCartesianToShoulderOriginCartesian.vi"("ArmPositionIn"=w103, "RobotDimensions"=w102) -> ("ArmPositionRelativeToShoulder"=w104:T6)
        n29 = call "ArmGoToPosition.vi"("RobotConfig"=T14 {"Motors"={"DriveRightPrimary"={"CAN Address"=3, "Invert"=FALSE, "InvertSensor"=FALSE, "Unit Conversion Factor"=0.0, "Brake Mode"=enum."Override to Brake", "Reverse Limt Switch Mode"=enum."Normally Closed", "Forward Limt Swith Mode"=enum."Normally Closed", "PWM Channel"=enum."Invalid", "Motor Controller Type"=enum."Talon SRX", "Peak Current (A)"=0, "Continuos Current (A)"=0, "Peak Duration (ms)"=0, "Current Limit Enable"=FALSE}, "DriveRightSecondary"={"CAN Address"=2, "Invert"=FALSE, "InvertSensor"=FALSE, "Unit Conversion Factor"=0.0, "Brake Mode"=enum."Override to Brake", "Reverse Limt Switch Mode"=enum."Normally Closed", "Forward Limt Swith Mode"=enum."Normally Closed", "PWM Channel"=enum."Invalid", "Motor Controller Type"=enum."Talon SRX", "Peak Current (A)"=0, "Continuos Current (A)"=0, "Peak Duration (ms)"=0, "Current Limit Enable"=FALSE}, "DriveLeftPrimary"={"CAN Address"=1, "Invert"=FALSE, "InvertSensor"=FALSE, "Unit Conversion Factor"=0.0, "Brake Mode"=enum."Override to Brake", "Reverse Limt Switch Mode"=enum."Normally Closed", "Forward Limt Swith Mode"=enum."Normally Closed", "PWM Channel"=enum."Invalid", "Motor Controller Type"=enum."Talon SRX", "Peak Current (A)"=0, "Continuos Current (A)"=0, "Peak Duration (ms)"=0, "Current Limit Enable"=FALSE}, "DriveLeftSecondary"={"CAN Address"=4, "Invert"=FALSE, "InvertSensor"=FALSE, "Unit Conversion Factor"=0.0, "Brake Mode"=enum."Override to Brake", "Reverse Limt Switch Mode"=enum."Normally Closed", "Forward Limt Swith Mode"=enum."Normally Closed", "PWM Channel"=enum."Invalid", "Motor Controller Type"=enum."Talon SRX", "Peak Current (A)"=0, "Continuos Current (A)"=0, "Peak Duration (ms)"=0, "Current Limit Enable"=FALSE}, "RearClimb"={"CAN Address"=8, "Invert"=FALSE, "InvertSensor"=FALSE, "Unit Conversion Factor"=0.0, "Brake Mode"=enum."Override to Brake", "Reverse Limt Switch Mode"=enum."Normally Closed", "Forward Limt Swith Mode"=enum."Normally Closed", "PWM Channel"=enum."Invalid", "Motor Controller Type"=enum."Talon SRX", "Peak Current (A)"=0, "Continuos Current (A)"=0, "Peak Duration (ms)"=0, "Current Limit Enable"=FALSE}, "Front Climb"={"CAN Address"=7, "Invert"=FALSE, "InvertSensor"=FALSE, "Unit Conversion Factor"=0.0, "Brake Mode"=enum."Override to Brake", "Reverse Limt Switch Mode"=enum."Normally Closed", "Forward Limt Swith Mode"=enum."Normally Closed", "PWM Channel"=enum."Invalid", "Motor Controller Type"=enum."Talon SRX", "Peak Current (A)"=0, "Continuos Current (A)"=0, "Peak Duration (ms)"=0, "Current Limit Enable"=FALSE}, "Climb Drive"={"CAN Address"=5, "Invert"=FALSE, "InvertSensor"=FALSE, "Unit Conversion Factor"=0.0, "Brake Mode"=enum."Override to Brake", "Reverse Limt Switch Mode"=enum."Normally Closed", "Forward Limt Swith Mode"=enum."Normally Closed", "PWM Channel"=enum."Invalid", "Motor Controller Type"=enum."Talon SRX", "Peak Current (A)"=0, "Continuos Current (A)"=0, "Peak Duration (ms)"=0, "Current Limit Enable"=FALSE}, "Shoulder1"={"CAN Address"=6, "Invert"=FALSE, "InvertSensor"=FALSE, "Unit Conversion Factor"=0.0, "Brake Mode"=enum."Override to Brake", "Reverse Limt Switch Mode"=enum."Normally Closed", "Forward Limt Swith Mode"=enum."Normally Closed", "PWM Channel"=enum."Invalid", "Motor Controller Type"=enum."Talon SRX", "Peak Current (A)"=0, "Continuos Current (A)"=0, "Peak Duration (ms)"=0, "Current Limit Enable"=FALSE}, "Shoulder2"={"CAN Address"=9, "Invert"=FALSE, "InvertSensor"=FALSE, "Unit Conversion Factor"=0.0, "Brake Mode"=enum."Override to Brake", "Reverse Limt Switch Mode"=enum."Normally Closed", "Forward Limt Swith Mode"=enum."Normally Closed", "PWM Channel"=enum."Invalid", "Motor Controller Type"=enum."Talon SRX", "Peak Current (A)"=0, "Continuos Current (A)"=0, "Peak Duration (ms)"=0, "Current Limit Enable"=FALSE}, "Wrist"={"CAN Address"=10, "Invert"=FALSE, "InvertSensor"=FALSE, "Unit Conversion Factor"=0.0, "Brake Mode"=enum."Override to Brake", "Reverse Limt Switch Mode"=enum."Disabled", "Forward Limt Swith Mode"=enum."Disabled", "PWM Channel"=enum."Invalid", "Motor Controller Type"=enum."Talon SRX", "Peak Current (A)"=0, "Continuos Current (A)"=0, "Peak Duration (ms)"=0, "Current Limit Enable"=FALSE}, "Extension"={"CAN Address"=11, "Invert"=FALSE, "InvertSensor"=FALSE, "Unit Conversion Factor"=0.0, "Brake Mode"=enum."Override to Brake", "Reverse Limt Switch Mode"=enum."Disabled", "Forward Limt Swith Mode"=enum."Disabled", "PWM Channel"=enum."Invalid", "Motor Controller Type"=enum."Talon SRX", "Peak Current (A)"=0, "Continuos Current (A)"=0, "Peak Duration (ms)"=0, "Current Limit Enable"=FALSE}, "CargoIntake"={"CAN Address"=0, "Invert"=FALSE, "InvertSensor"=FALSE, "Unit Conversion Factor"=1.0, "Brake Mode"=enum."Override to Brake", "Reverse Limt Switch Mode"=enum."Disabled", "Forward Limt Swith Mode"=enum."Normally Open", "PWM Channel"=enum."PWM 8", "Motor Controller Type"=enum."Talon SR", "Peak Current (A)"=0, "Continuos Current (A)"=0, "Peak Duration (ms)"=0, "Current Limit Enable"=FALSE}, "Intake2"={"CAN Address"=10, "Invert"=FALSE, "InvertSensor"=TRUE, "Unit Conversion Factor"=0.0, "Brake Mode"=enum."Override to Brake", "Reverse Limt Switch Mode"=enum."Normally Open", "Forward Limt Swith Mode"=enum."Normally Open", "PWM Channel"=enum."PWM 0", "Motor Controller Type"=enum."Disabled", "Peak Current (A)"=0, "Continuos Current (A)"=0, "Peak Duration (ms)"=0, "Current Limit Enable"=FALSE}}, "Sensors"={"IMU"={"Yaw Axis"=enum."Z", "SPI Bus"=enum."SPI MXP", "AHRS Algorithm"=enum."Complementary", "Calibration Time (s)"=3.0, "Calibrate On Open"=TRUE}, "HomingButton"={"DIOChannel"=enum."DIO 0", "Active Low"=FALSE}, "HomingLED_Green"={"DIOChannel"=enum."DIO 0", "Active Low"=FALSE}, "HomingLED_Yellow"={"DIOChannel"=enum."DIO 0", "Active Low"=FALSE}, "HomingLED_Red"={"DIOChannel"=enum."DIO 0", "Active Low"=FALSE}}, "PID"={"FrontClimb"={"P"=0.0, "I"=0.0, "D"=0.0, "F"=0.0, "IZone"=0.0}, "RearClimb"={"P"=0.0, "I"=0.0, "D"=0.0, "F"=0.0, "IZone"=0.0}, "ArmShoulder"={"P"=0.0, "I"=0.0, "D"=0.0, "F"=0.0, "IZone"=0.0}, "ArmExtend"={"P"=0.0, "I"=0.0, "D"=0.0, "F"=0.0, "IZone"=0.0}, "ArmWrist"={"P"=0.0, "I"=0.0, "D"=0.0, "F"=0.0, "IZone"=0.0}}, "Solenoids"={" Shifter"={"SolenoidChannel"=enum."Solenoid 3", "Invert"=FALSE}, "Hatch Grip"={"SolenoidChannel"=enum."Solenoid 0", "Invert"=FALSE}, "Hatch Extend"={"SolenoidChannel"=enum."Solenoid 1", "Invert"=FALSE}, "Manipulator Slide"={"SolenoidChannel"=enum."Solenoid 2", "Invert"=FALSE}, "Hatch Floor Intake"={"SolenoidChannel"=enum."Solenoid 0", "Invert"=FALSE}}, "Enable Compressor"=TRUE, "MotionMagic"={"FrontClimbExtend"={"CruiseVelocity"=0, "Acceleration"=0}, "RearClimbExtend"={"CruiseVelocity"=0, "Acceleration"=0}, "FrontClimbRetract"={"CruiseVelocity"=0, "Acceleration"=0}, "RearClimbRetract"={"CruiseVelocity"=0, "Acceleration"=0}}, "RobotDimensions"={"Length (in)"=0.0, "Shoulder Height (in)"=0.0, "Frame Height (in)"=0.0, "Arm Center to Front of Robot (in)"=0.0, "Arm Min Extension (in)"=0.0, "Arm Max Extension (in)"=0.0, "Cargo Intake Loop Length (in)"=0.0, "Cargo Intake Loop Width (in)"=0.0, "Cargo Intake Loop Offset (in)"=0.0, "Cargo Intake Loop Angle (rad)"=0.0}, "Arm Home Position"={"Radius (in)"=0.0, "ShoulderAngle (rad)"=0.0, "WristAngle (rad)"=0.0}, "Climb Home Position"={"Back Climb"=0.0, "Front Climb"=0.0}, "Climb Positions"={"Retract"=0.0, "Level 2"=0.0, "Level 3"=0.0}}, "ArmPlanRequest"=w118, "Arm min Extension (in)"=w112, "Arm max Extension (in)"=w111, "Game Piece Position"=w109, "Avoidance Polygon"=w108, "RobotMotors"=T31 {"DriveRightPrimary"={"DeviceStatus"={"status"=FALSE, "code"=0, "source"=""}, "Type"=enum."PWM", "PWM"={"PWM Channel"=enum."PWM 1", "DeadBand"={"Name"="", "maxPositivePwm"=0, "minPositivePwm"=0, "centerPwm"=0, "maxNegativePwm"=0, "minNegativePwm"=0, "angularRange"=0}}, "CAN"={"Device Number"=0, "SetOutput VI Ref"=variant(enum8{"Percent VBus", "Current", "Speed", "Position", "Voltage"} enum."Percent VBus"), "GetOutput VI Ref"=variant(refnum<k1> refnum), "Enable VI Ref"=variant(dbl 12.0), "Disable VI Ref"=variant(enum8{"Percent VBus", "Speed", "Position", "Slave", "Unchanged / Invalid", "Voltage Compensation", "Current", "Motion Profile"} enum."Percent VBus"), "Data"=variant}, "Invert"=FALSE, "DIO PWM"={"PWM \"Enable\" Channel"=enum."Invalid", "DIOChannel"=enum."Invalid", "PWM Rate"=0.0}}, "DriveRightSecondary"={"DeviceStatus"={"status"=FALSE, "code"=0, "source"=""}, "Type"=enum."PWM", "PWM"={"PWM Channel"=enum."PWM 1", "DeadBand"={"Name"="", "maxPositivePwm"=0, "minPositivePwm"=0, "centerPwm"=0, "maxNegativePwm"=0, "minNegativePwm"=0, "angularRange"=0}}, "CAN"={"Device Number"=0, "SetOutput VI Ref"=variant(enum8{"Percent VBus", "Current", "Speed", "Position", "Voltage"} enum."Percent VBus"), "GetOutput VI Ref"=variant(refnum<k1> refnum), "Enable VI Ref"=variant(dbl 12.0), "Disable VI Ref"=variant(enum8{"Percent VBus", "Speed", "Position", "Slave", "Unchanged / Invalid", "Voltage Compensation", "Current", "Motion Profile"} enum."Percent VBus"), "Data"=variant}, "Invert"=FALSE, "DIO PWM"={"PWM \"Enable\" Channel"=enum."Invalid", "DIOChannel"=enum."Invalid", "PWM Rate"=0.0}}, "DriveLeftPrimary"={"DeviceStatus"={"status"=FALSE, "code"=0, "source"=""}, "Type"=enum."PWM", "PWM"={"PWM Channel"=enum."PWM 1", "DeadBand"={"Name"="", "maxPositivePwm"=0, "minPositivePwm"=0, "centerPwm"=0, "maxNegativePwm"=0, "minNegativePwm"=0, "angularRange"=0}}, "CAN"={"Device Number"=0, "SetOutput VI Ref"=variant(enum8{"Percent VBus", "Current", "Speed", "Position", "Voltage"} enum."Percent VBus"), "GetOutput VI Ref"=variant(refnum<k1> refnum), "Enable VI Ref"=variant(dbl 12.0), "Disable VI Ref"=variant(enum8{"Percent VBus", "Speed", "Position", "Slave", "Unchanged / Invalid", "Voltage Compensation", "Current", "Motion Profile"} enum."Percent VBus"), "Data"=variant}, "Invert"=FALSE, "DIO PWM"={"PWM \"Enable\" Channel"=enum."Invalid", "DIOChannel"=enum."Invalid", "PWM Rate"=0.0}}, "DriveLeftSecondary"={"DeviceStatus"={"status"=FALSE, "code"=0, "source"=""}, "Type"=enum."PWM", "PWM"={"PWM Channel"=enum."PWM 1", "DeadBand"={"Name"="", "maxPositivePwm"=0, "minPositivePwm"=0, "centerPwm"=0, "maxNegativePwm"=0, "minNegativePwm"=0, "angularRange"=0}}, "CAN"={"Device Number"=0, "SetOutput VI Ref"=variant(enum8{"Percent VBus", "Current", "Speed", "Position", "Voltage"} enum."Percent VBus"), "GetOutput VI Ref"=variant(refnum<k1> refnum), "Enable VI Ref"=variant(dbl 12.0), "Disable VI Ref"=variant(enum8{"Percent VBus", "Speed", "Position", "Slave", "Unchanged / Invalid", "Voltage Compensation", "Current", "Motion Profile"} enum."Percent VBus"), "Data"=variant}, "Invert"=FALSE, "DIO PWM"={"PWM \"Enable\" Channel"=enum."Invalid", "DIOChannel"=enum."Invalid", "PWM Rate"=0.0}}, " RearClimb"={"DeviceStatus"={"status"=FALSE, "code"=0, "source"=""}, "Type"=enum."PWM", "PWM"={"PWM Channel"=enum."PWM 1", "DeadBand"={"Name"="", "maxPositivePwm"=0, "minPositivePwm"=0, "centerPwm"=0, "maxNegativePwm"=0, "minNegativePwm"=0, "angularRange"=0}}, "CAN"={"Device Number"=0, "SetOutput VI Ref"=variant(enum8{"Percent VBus", "Current", "Speed", "Position", "Voltage"} enum."Percent VBus"), "GetOutput VI Ref"=variant(refnum<k1> refnum), "Enable VI Ref"=variant(dbl 12.0), "Disable VI Ref"=variant(enum8{"Percent VBus", "Speed", "Position", "Slave", "Unchanged / Invalid", "Voltage Compensation", "Current", "Motion Profile"} enum."Percent VBus"), "Data"=variant}, "Invert"=FALSE, "DIO PWM"={"PWM \"Enable\" Channel"=enum."Invalid", "DIOChannel"=enum."Invalid", "PWM Rate"=0.0}}, "FrontClimb"={"DeviceStatus"={"status"=FALSE, "code"=0, "source"=""}, "Type"=enum."PWM", "PWM"={"PWM Channel"=enum."PWM 1", "DeadBand"={"Name"="", "maxPositivePwm"=0, "minPositivePwm"=0, "centerPwm"=0, "maxNegativePwm"=0, "minNegativePwm"=0, "angularRange"=0}}, "CAN"={"Device Number"=0, "SetOutput VI Ref"=variant(enum8{"Percent VBus", "Current", "Speed", "Position", "Voltage"} enum."Percent VBus"), "GetOutput VI Ref"=variant(refnum<k1> refnum), "Enable VI Ref"=variant(dbl 12.0), "Disable VI Ref"=variant(enum8{"Percent VBus", "Speed", "Position", "Slave", "Unchanged / Invalid", "Voltage Compensation", "Current", "Motion Profile"} enum."Percent VBus"), "Data"=variant}, "Invert"=FALSE, "DIO PWM"={"PWM \"Enable\" Channel"=enum."Invalid", "DIOChannel"=enum."Invalid", "PWM Rate"=0.0}}, "ClimbDrive"={"DeviceStatus"={"status"=FALSE, "code"=0, "source"=""}, "Type"=enum."PWM", "PWM"={"PWM Channel"=enum."PWM 1", "DeadBand"={"Name"="", "maxPositivePwm"=0, "minPositivePwm"=0, "centerPwm"=0, "maxNegativePwm"=0, "minNegativePwm"=0, "angularRange"=0}}, "CAN"={"Device Number"=0, "SetOutput VI Ref"=variant(enum8{"Percent VBus", "Current", "Speed", "Position", "Voltage"} enum."Percent VBus"), "GetOutput VI Ref"=variant(refnum<k1> refnum), "Enable VI Ref"=variant(dbl 12.0), "Disable VI Ref"=variant(enum8{"Percent VBus", "Speed", "Position", "Slave", "Unchanged / Invalid", "Voltage Compensation", "Current", "Motion Profile"} enum."Percent VBus"), "Data"=variant}, "Invert"=FALSE, "DIO PWM"={"PWM \"Enable\" Channel"=enum."Invalid", "DIOChannel"=enum."Invalid", "PWM Rate"=0.0}}, "Shoulder2"={"DeviceStatus"={"status"=FALSE, "code"=0, "source"=""}, "Type"=enum."PWM", "PWM"={"PWM Channel"=enum."PWM 1", "DeadBand"={"Name"="", "maxPositivePwm"=0, "minPositivePwm"=0, "centerPwm"=0, "maxNegativePwm"=0, "minNegativePwm"=0, "angularRange"=0}}, "CAN"={"Device Number"=0, "SetOutput VI Ref"=variant(enum8{"Percent VBus", "Current", "Speed", "Position", "Voltage"} enum."Percent VBus"), "GetOutput VI Ref"=variant(refnum<k1> refnum), "Enable VI Ref"=variant(dbl 12.0), "Disable VI Ref"=variant(enum8{"Percent VBus", "Speed", "Position", "Slave", "Unchanged / Invalid", "Voltage Compensation", "Current", "Motion Profile"} enum."Percent VBus"), "Data"=variant}, "Invert"=FALSE, "DIO PWM"={"PWM \"Enable\" Channel"=enum."Invalid", "DIOChannel"=enum."Invalid", "PWM Rate"=0.0}}, "Shoulder1 "={"DeviceStatus"={"status"=FALSE, "code"=0, "source"=""}, "Type"=enum."PWM", "PWM"={"PWM Channel"=enum."PWM 1", "DeadBand"={"Name"="", "maxPositivePwm"=0, "minPositivePwm"=0, "centerPwm"=0, "maxNegativePwm"=0, "minNegativePwm"=0, "angularRange"=0}}, "CAN"={"Device Number"=0, "SetOutput VI Ref"=variant(enum8{"Percent VBus", "Current", "Speed", "Position", "Voltage"} enum."Percent VBus"), "GetOutput VI Ref"=variant(refnum<k1> refnum), "Enable VI Ref"=variant(dbl 12.0), "Disable VI Ref"=variant(enum8{"Percent VBus", "Speed", "Position", "Slave", "Unchanged / Invalid", "Voltage Compensation", "Current", "Motion Profile"} enum."Percent VBus"), "Data"=variant}, "Invert"=FALSE, "DIO PWM"={"PWM \"Enable\" Channel"=enum."Invalid", "DIOChannel"=enum."Invalid", "PWM Rate"=0.0}}, "Wrist"={"DeviceStatus"={"status"=FALSE, "code"=0, "source"=""}, "Type"=enum."PWM", "PWM"={"PWM Channel"=enum."PWM 1", "DeadBand"={"Name"="", "maxPositivePwm"=0, "minPositivePwm"=0, "centerPwm"=0, "maxNegativePwm"=0, "minNegativePwm"=0, "angularRange"=0}}, "CAN"={"Device Number"=0, "SetOutput VI Ref"=variant(enum8{"Percent VBus", "Current", "Speed", "Position", "Voltage"} enum."Percent VBus"), "GetOutput VI Ref"=variant(refnum<k1> refnum), "Enable VI Ref"=variant(dbl 12.0), "Disable VI Ref"=variant(enum8{"Percent VBus", "Speed", "Position", "Slave", "Unchanged / Invalid", "Voltage Compensation", "Current", "Motion Profile"} enum."Percent VBus"), "Data"=variant}, "Invert"=FALSE, "DIO PWM"={"PWM \"Enable\" Channel"=enum."Invalid", "DIOChannel"=enum."Invalid", "PWM Rate"=0.0}}, "Extension"={"DeviceStatus"={"status"=FALSE, "code"=0, "source"=""}, "Type"=enum."PWM", "PWM"={"PWM Channel"=enum."PWM 1", "DeadBand"={"Name"="", "maxPositivePwm"=0, "minPositivePwm"=0, "centerPwm"=0, "maxNegativePwm"=0, "minNegativePwm"=0, "angularRange"=0}}, "CAN"={"Device Number"=0, "SetOutput VI Ref"=variant(enum8{"Percent VBus", "Current", "Speed", "Position", "Voltage"} enum."Percent VBus"), "GetOutput VI Ref"=variant(refnum<k1> refnum), "Enable VI Ref"=variant(dbl 12.0), "Disable VI Ref"=variant(enum8{"Percent VBus", "Speed", "Position", "Slave", "Unchanged / Invalid", "Voltage Compensation", "Current", "Motion Profile"} enum."Percent VBus"), "Data"=variant}, "Invert"=FALSE, "DIO PWM"={"PWM \"Enable\" Channel"=enum."Invalid", "DIOChannel"=enum."Invalid", "PWM Rate"=0.0}}, "CargoIntake"={"DeviceStatus"={"status"=FALSE, "code"=0, "source"=""}, "Type"=enum."PWM", "PWM"={"PWM Channel"=enum."PWM 1", "DeadBand"={"Name"="", "maxPositivePwm"=0, "minPositivePwm"=0, "centerPwm"=0, "maxNegativePwm"=0, "minNegativePwm"=0, "angularRange"=0}}, "CAN"={"Device Number"=0, "SetOutput VI Ref"=variant(enum8{"Percent VBus", "Current", "Speed", "Position", "Voltage"} enum."Percent VBus"), "GetOutput VI Ref"=variant(refnum<k1> refnum), "Enable VI Ref"=variant(dbl 12.0), "Disable VI Ref"=variant(enum8{"Percent VBus", "Speed", "Position", "Slave", "Unchanged / Invalid", "Voltage Compensation", "Current", "Motion Profile"} enum."Percent VBus"), "Data"=variant}, "Invert"=FALSE, "DIO PWM"={"PWM \"Enable\" Channel"=enum."Invalid", "DIOChannel"=enum."Invalid", "PWM Rate"=0.0}}, "Intake2"={"DeviceStatus"={"status"=FALSE, "code"=0, "source"=""}, "Type"=enum."PWM", "PWM"={"PWM Channel"=enum."PWM 1", "DeadBand"={"Name"="", "maxPositivePwm"=0, "minPositivePwm"=0, "centerPwm"=0, "maxNegativePwm"=0, "minNegativePwm"=0, "angularRange"=0}}, "CAN"={"Device Number"=0, "SetOutput VI Ref"=variant(enum8{"Percent VBus", "Current", "Speed", "Position", "Voltage"} enum."Percent VBus"), "GetOutput VI Ref"=variant(refnum<k1> refnum), "Enable VI Ref"=variant(dbl 12.0), "Disable VI Ref"=variant(enum8{"Percent VBus", "Speed", "Position", "Slave", "Unchanged / Invalid", "Voltage Compensation", "Current", "Motion Profile"} enum."Percent VBus"), "Data"=variant}, "Invert"=FALSE, "DIO PWM"={"PWM \"Enable\" Channel"=enum."Invalid", "DIOChannel"=enum."Invalid", "PWM Rate"=0.0}}}, "MotionProfileGeneratorParameters"=w114, "Arm Pass Through Params"=w113, "RobotDimensions"=w110, "TestMode"=TRUE, "Test_ArmAbsolutePose"=w104) -> ("ArmPlanResponse"=w106:T38)  [unwired: 7 in]
        n30 = Tick Count (ms)() -> (millisecond timer value=w105:u32)
      }
    }
    n31 = feedback-in #2(w37) -> ()
    n32 = feedback-in #3(w41) -> ()
    n33 = Unbundle By Name(w41) -> ("ShoulderTrajectory"=w44:T13[])
    n34 = Subtract(x=w38, y=w37) -> (x-y=w35:u32)
    n35 = Array Size(array=w44) -> (size(s)=w43:i32)
    n36 = call "DrawCircle.vi"("YCenter"=w50, "XCenter"=w47, "Radius"=w54) -> ("Points"=w23:cluster{"X":dbl[], "Y":dbl[]})  [unwired: 1 in]
    n37 = call "DrawCircle.vi"("YCenter"=w50, "XCenter"=w47, "Radius"=w53) -> ("Points"=w24:cluster{"X":dbl[], "Y":dbl[]})  [unwired: 1 in]
    n38 = call "DrawPolygon2D.vi"("Polygon"=w55) -> ("XYPlot"=w25:cluster{dbl[], dbl[]})
    n39 = Equal To 0?(x=w43) -> (x = 0?=w42:bool)
    n40 = case shown="True" w42 {
      tunnel: w41 -> [w97 _]
      tunnel: w27 -> [_ w99]
      tunnel: [w97 w98] -> w11
      frame False {
      }
      frame True {
        n41 = call "ArmPositionToZeroLengthPlanResponse.vi"("Position"=w99) -> ("ArmPlanResponse"=w98:T38)
      }
    }
    n42 = Unbundle By Name(w11) -> ("PlanTime (ms)"=w36:u32)
    n43 = Unbundle By Name(w11) -> ("ShoulderTrajectory"=w10:T13[], "ExtendTrajectory"=w9:T13[], "WristTrajectory"=w8:T13[])
    n44 = local read "Arm MotionProfileParams"() -> (w3:T7)
    n45 = call "ArmPlanToPath.vi"("ArmPlanResponse"=w11) -> ("Path"=w5:T29[])
    n46 = Divide(x=w35, y=w36) -> (x/y=w34:dbl)
    n47 = In Range and Coerce(upper limit=1.0, x=w34, lower limit=0.0) -> (coerced(x)=w33:dbl)  [unwired: 1 out]
    n48 = Unbundle By Name(w3) -> ("Trajectory Point Interval (ms)"=w2:T8)
    n49 = call "CoordinateConvert_ArmToCartesian_Arrays.vi"("ArmCoordinates"=w5) -> ("XYPoints"=w21:T6[])
    n50 = call "ArmPathLength.vi"("ArmPathIn"=w5) -> ("IndexedPathLength"=w7:dbl[])  [unwired: 2 in, 2 out]
    n51 = call "CoordinateConvert_ShoulderOriginCartesianToWorldCartesian_Array.vi"("ArmPositionRelativeToShoulderIn"=w21, "RobotDimensions"=w22) -> ("ArmAbsolutePosition"=w18:T6[])
    n52 = call "PlotMotionProfile.vi"("Trajectory Points"=w10) -> ("MotionProfileGraph"=→"Arm Shoulder":T39)
    n53 = call "PlotMotionProfile.vi"("Trajectory Points"=w9) -> ("MotionProfileGraph"=→"Arm Extension":T39)
    n54 = call "PlotMotionProfile.vi"("Trajectory Points"=w8) -> ("MotionProfileGraph"=→"Arm Wrist":T39)
    n55 = for {
      tunnel: w18 -> [w96] mode=indexing
      tunnel: [w95] -> w20 mode=indexing
      tunnel: [w94] -> w19 mode=indexing
      n56 = Unbundle By Name(w96) -> ("X (in)"=w95:dbl, "Y (in)"=w94:dbl)
    }
    n57 = Index Array(array=w7) -> (element=w6:dbl)  [unwired: 1 in]
    n58 = Bundle(w20, w19) -> (w17:cluster{dbl[], dbl[]})  [unwired: 1 in]
    n59 = for {
      tunnel: [w92] -> w4 mode=indexing
      tunnel: w7 -> [w91] mode=indexing
      tunnel: w2 -> [w89]
      shift-right: [w91] -> _
      shift-left: w6 -> [w90]
      n60 = Subtract(x=w91, y=w90) -> (x-y=w87:dbl)
      n61 = Divide(x=w89, y=1000) -> (x/y=w86:dbl)
      n62 = Divide(x=w87, y=w86) -> (x/y=w85:dbl)
      n63 = Bundle By Name(cluster=T13 {"Position "=0.0, "Velocity "=0.0, "Time (ms)"=0, "Last Point"=FALSE} ("trajectory point"), "Position"=w91, "Velocity"=w85, "Time (ms)"=w89) -> (w92:T13)
    }
    n64 = call "InteractiveDrawArmPath.vi"("PathPercent"=w33, "RobotDimensions"=w22, "AvoidancePolygon"=w25, "MaxRadiusCircle"=w24, "MinRadiusCircle"=w23, "Path"=w5) -> ("RawArmPosition"=w56:T6, "Arm Position"=→"Arm Position":cluster{"X":dbl[], "Y":dbl[]}[])  [unwired: 4 in]
    n65 = feedback-in #4(w56) -> ()
    n66 = Build Array(w23, w24, w25, w17) -> (→"Path":cluster{"X":dbl[], "Y":dbl[]}[])
    n67 = call "PlotMotionProfile.vi"("Trajectory Points"=w4) -> ("MotionProfileGraph"=→"Overall Motion":T39)
    n68 = Wait (ms)(milliseconds to wait=u32 10) -> ()  [unwired: 1 out]
  }
